vi "Make 2D Voltage Calibration Plots.vi"() -> ()   [LabVIEW 2019]
uses:
  <vilib>/Utility/file.llb/Read Delimited Spreadsheet (I64).vi
  <vilib>/Utility/file.llb/Write Delimited Spreadsheet (I64).vi
panel:
  out "Mask B Voltage vs. Mask A Voltage":i64[][](graph)
  in  "Pixel to Plot":i32
  in  "Pixel Data":path
  in  "Folder to save Pixel data":path
  in  "Starting Pixel":dbl
  in  "Starting Mask B Voltage":dbl
  in  "Ending Mask B Voltage":dbl
  in  "Current Mask B Voltage":dbl
  in  "Step Mask B Voltage":dbl
  in  "Generate Files (Px vs. Voltage)":bool
  in  "Ending Pixel":dbl
  in  "Current Pixel":dbl
  in  "Step":dbl
  in  "Folder of .txt 1D Calibration Files":path
  in  "Plot":bool
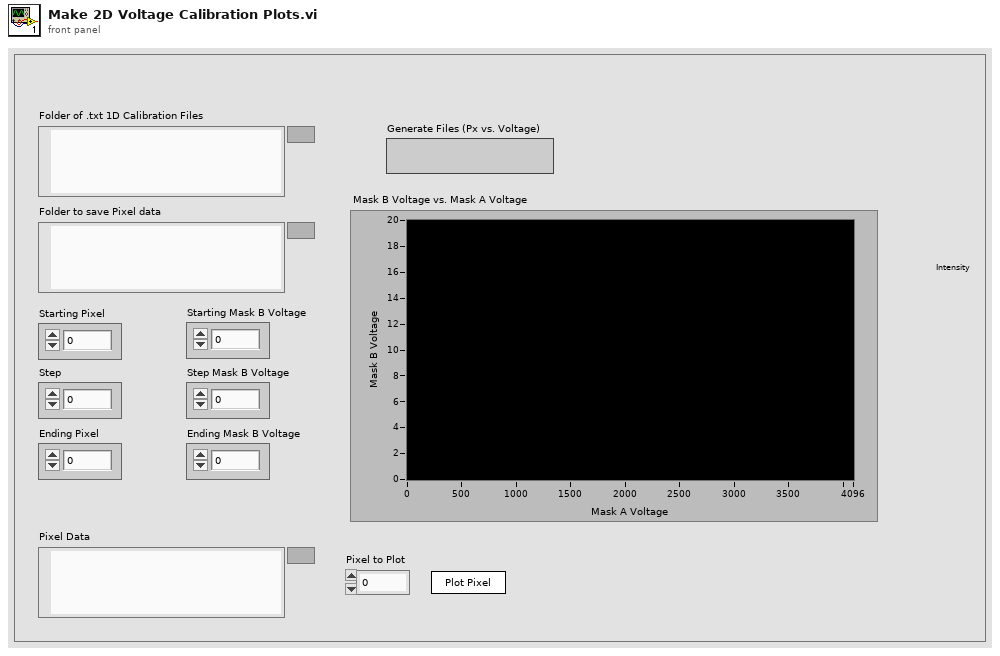
[diagram p1: front panel]
types:
  T1 = enum32{"Invalid", "Standard", "Closed", "Hidden", "Minimized", "Maximized"}
  T2 = enum32{"invalid app kind", "Development System", "Run Time System", "Student Edition", "Embedded LabVIEW", "Evaluation", "Custom"}
  T3 = enum16{"open", "replace", "create", "open or create", "replace or create", "replace or create with confirmation"}
  T4 = cluster{"Core":cluster{"Current VI Reference":refnum<vi>, "Close Panel on Exit?":bool}, "Starting Pixel":dbl, "Step":dbl, "Ending Pixel":dbl, "Current Pixel":dbl, "Starting Mask B Voltage":dbl, "Step Mask B Voltage":dbl, "Ending Mask B Voltage":dbl, "Current Mask B Voltage":dbl}
  T5 = cluster{"Current VI Reference":refnum<vi>, "Close Panel on Exit?":bool}
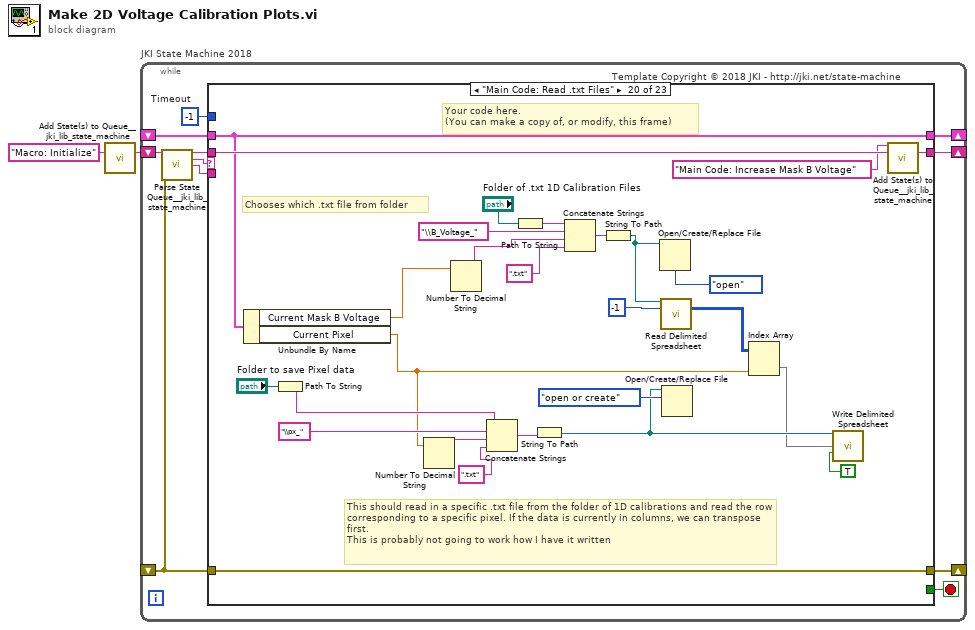
[diagram p0: block diagram]
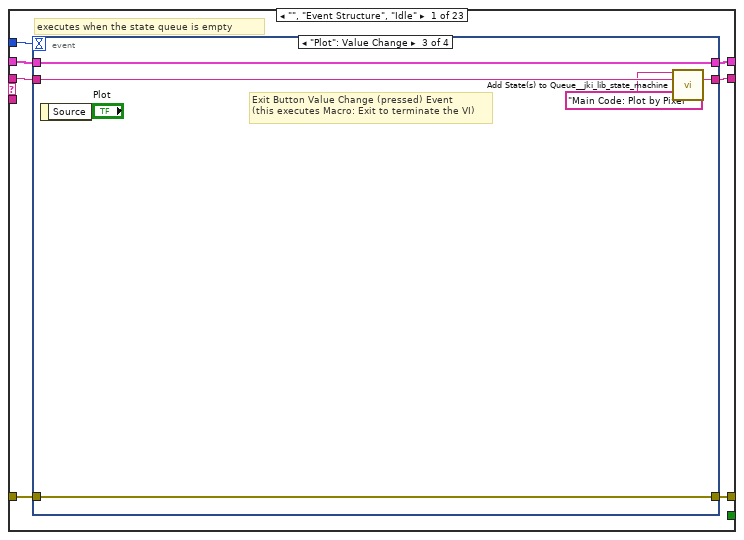
[diagram p2: hidden frame]
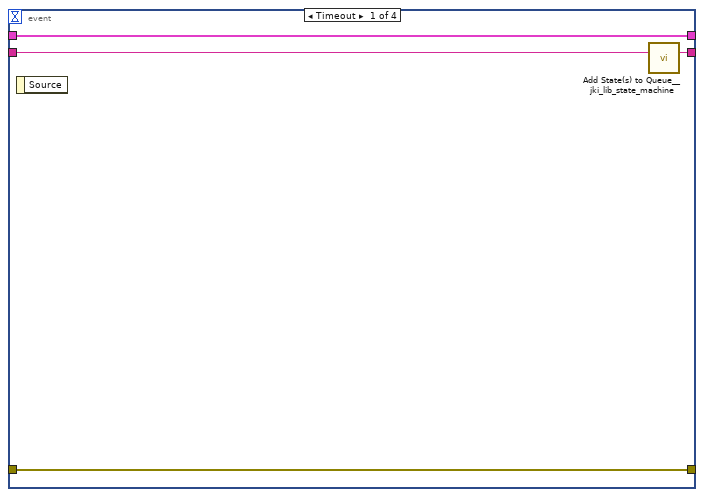
[diagram p3: hidden frame]
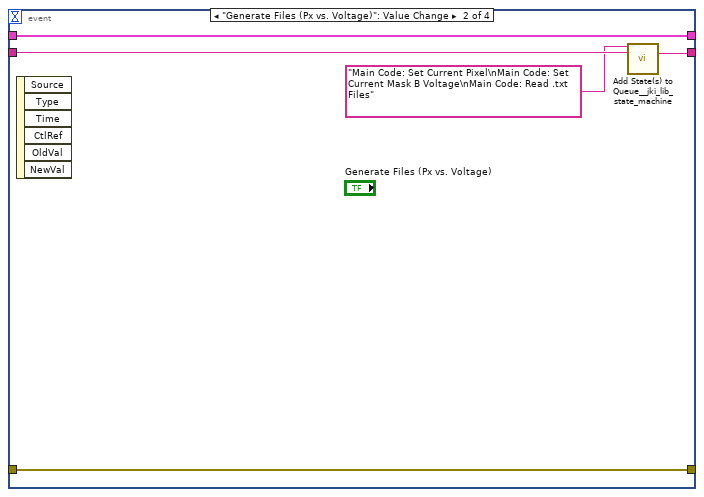
[diagram p4: hidden frame]
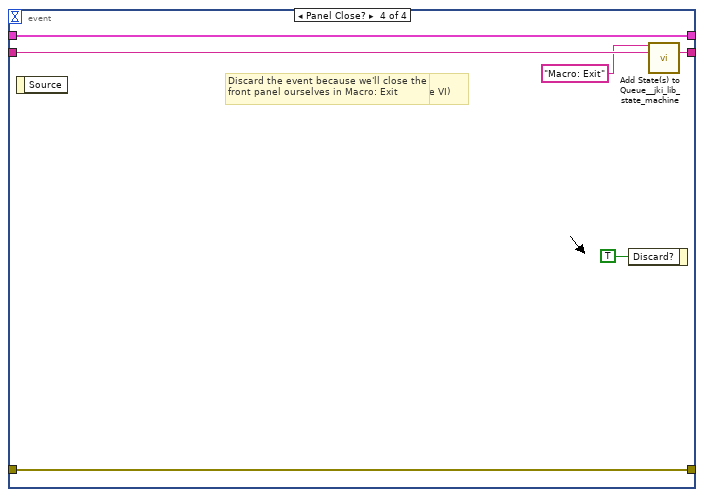
[diagram p5: hidden frame]
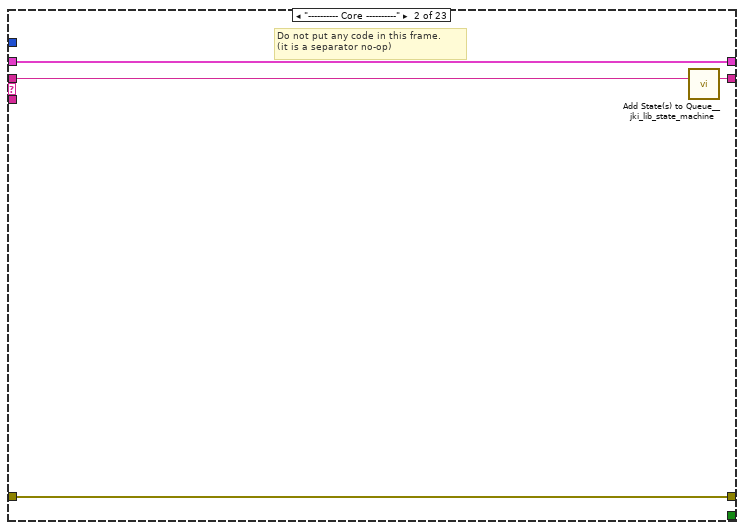
[diagram p6: hidden frame]
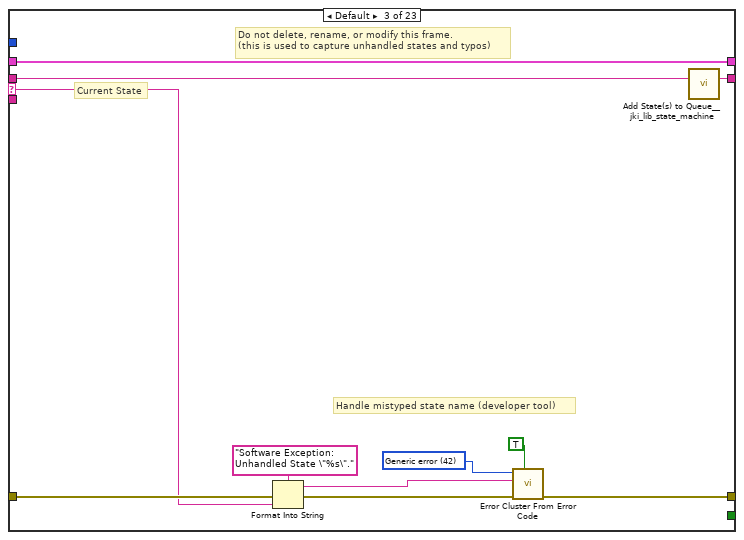
[diagram p7: hidden frame]
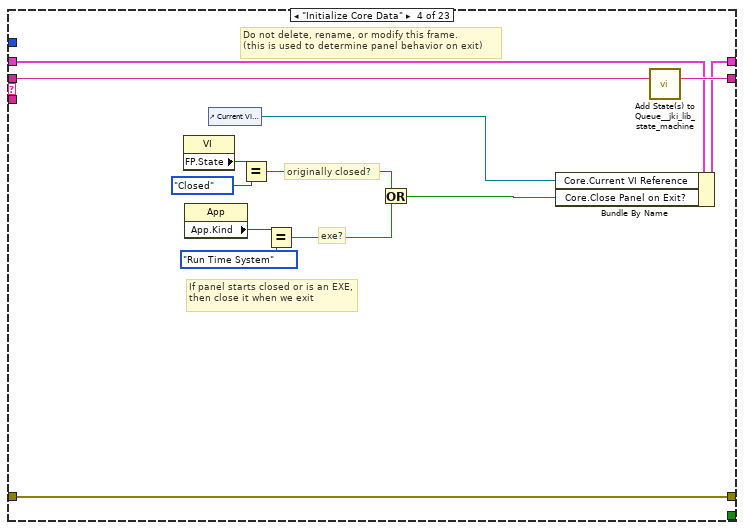
[diagram p8: hidden frame]
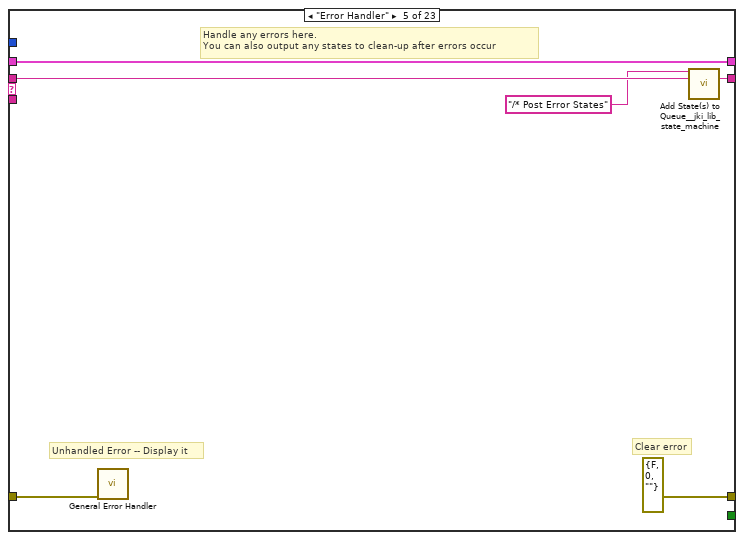
[diagram p9: hidden frame]
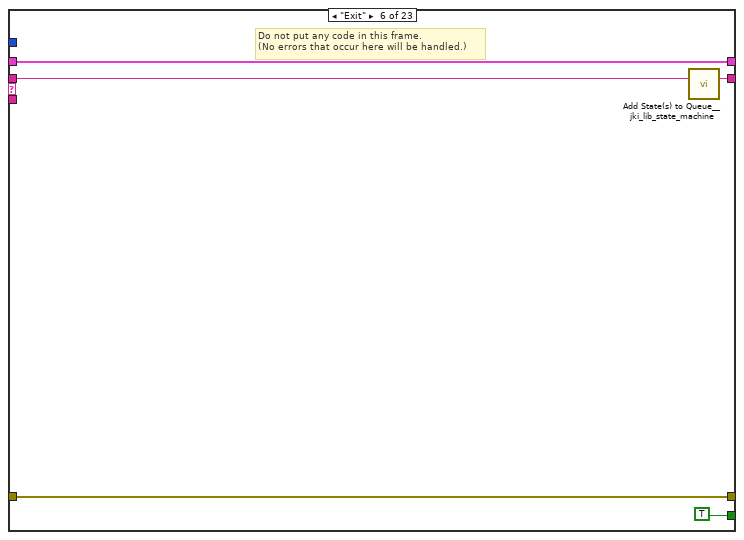
[diagram p10: hidden frame]
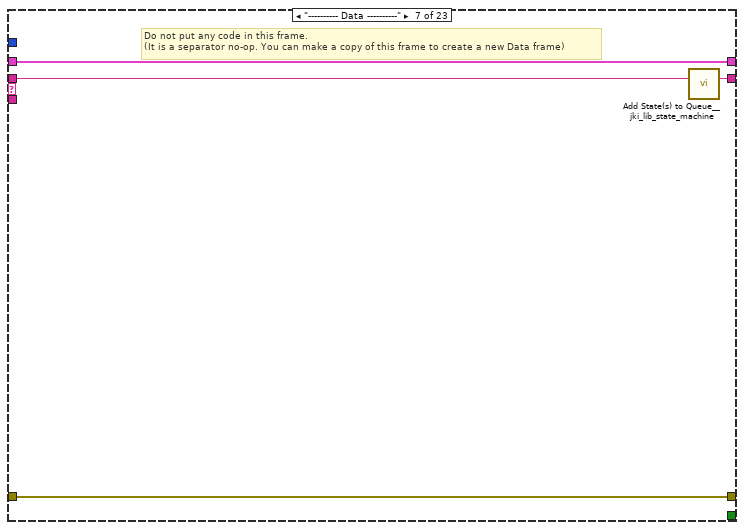
[diagram p11: hidden frame]
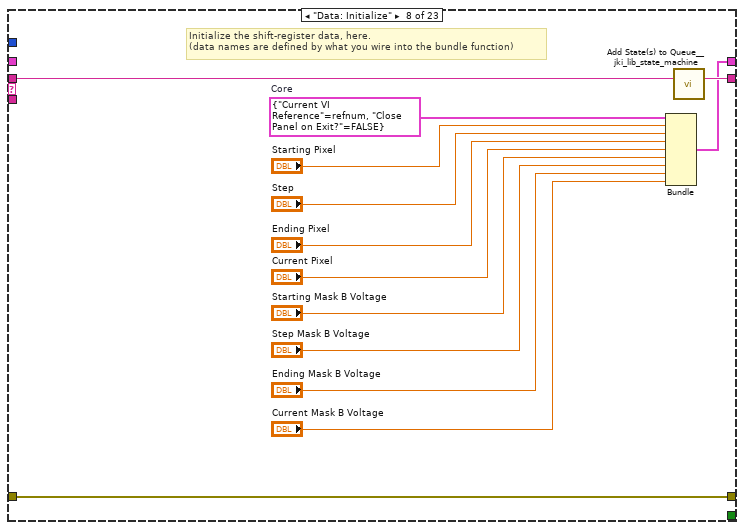
[diagram p12: hidden frame]
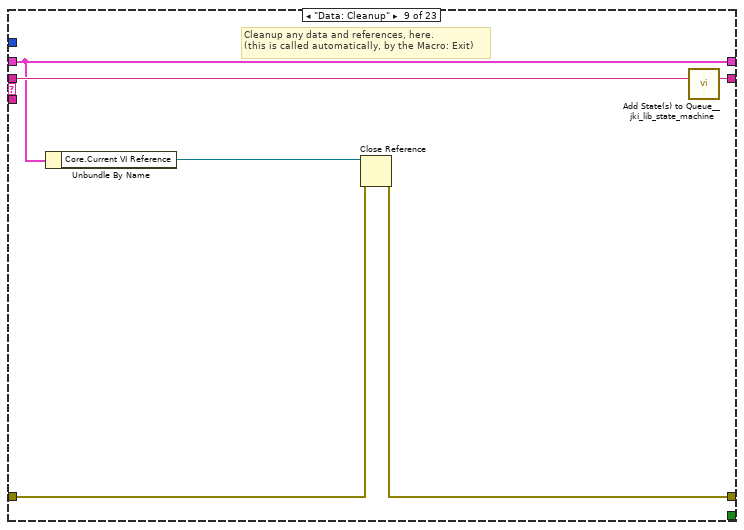
[diagram p13: hidden frame]
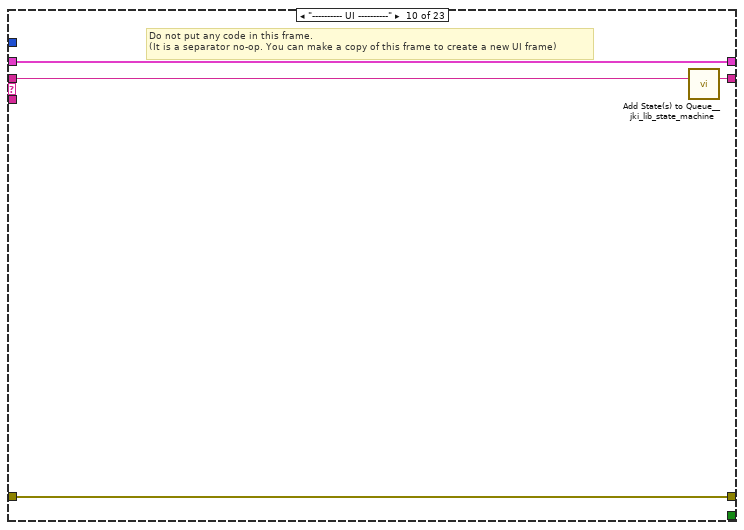
[diagram p14: hidden frame]
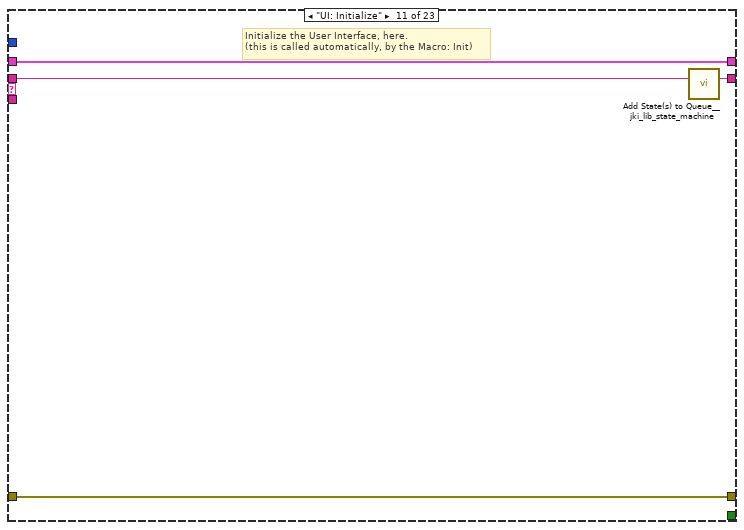
[diagram p15: hidden frame]
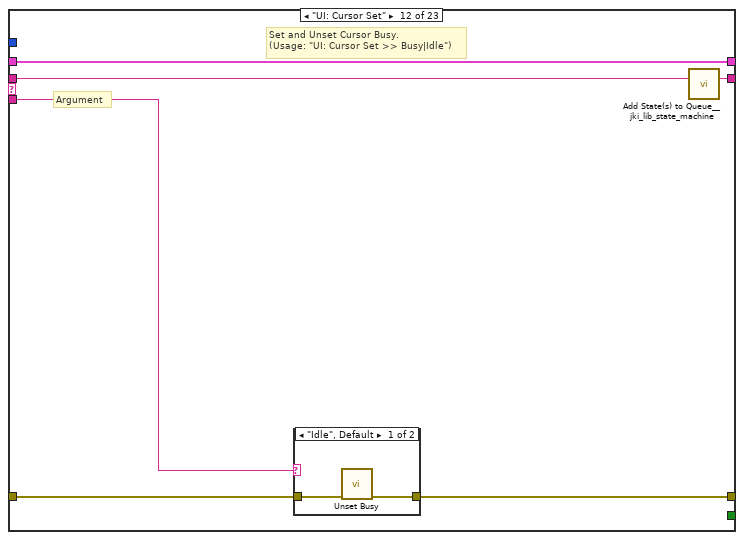
[diagram p16: hidden frame]
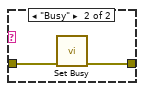
[diagram p17: hidden frame]
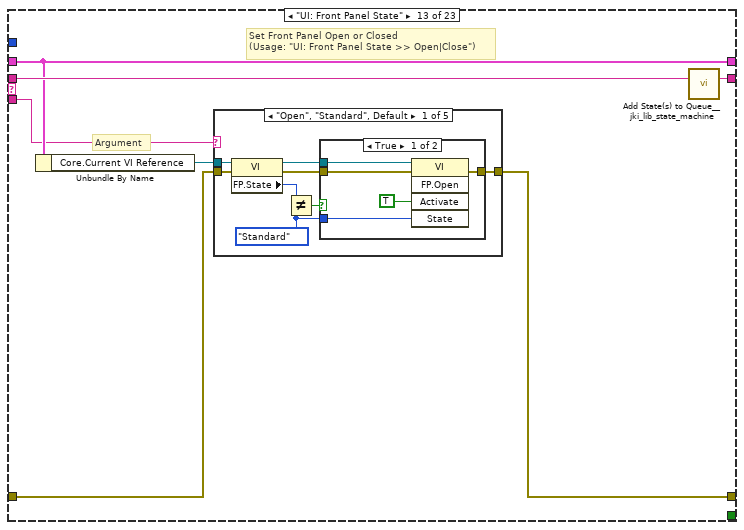
[diagram p18: hidden frame]
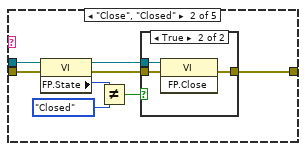
[diagram p20: hidden frame]
diagram:
  n1 = call <vilib>:"Add State(s) to Queue__jki_lib_state_machine.vi"("State(s) in (\"\")"="Macro: Initialize") -> ("States Out"=w2:string)  [unwired: 14 in]
  n2 = while "JKI State Machine 2018" {
    shift-right: [w6] -> _
    shift-left: _ -> [w5]
    shift-right: [w9] -> _
    shift-left: _ -> [w3]
    shift-right: [w8] -> _
    shift-left: w2 -> [w10]
    stop <- w7 stop-if-true
    w4 = -1  # Timeout
    # "Template Copyright © 2018 JKI - http://jki.net/state-machine"
    n3 = call <vilib>:"Parse State Queue__jki_lib_state_machine.vi"("State Queue"=w10, "Error In (no error)"=w3) -> ("Remaining States"=w12:string, "Current State"=w13:string, "Arguments"=w11:string)  [unwired: 11 in]
    n4 = case shown="\"Main Code: Read .txt Files\"" w13 {
      selector: w13 -> [_ _ w45 _ _ _ _ _ _ _ _ _ _ _ _ _ _ _ _ _ _ _ _]
      tunnel: w12 -> [w20 w44 w49 w68 w74 w79 w83 w96 w102 w106 w110 w116 w127 w196 w201 w211 w215 w221 w227 w254 w265 w285 w310]
      tunnel: w11 -> [_ _ _ _ _ _ _ _ _ _ _ w111 w121 _ _ _ _ _ _ _ _ _ _]
      tunnel: w5 -> [w18 w41 w47 w61 w71 w77 w80 _ w97 w103 w108 w114 w123 w193 w198 w208 w212 w218 w224 w243 w257 w278 w307]
      tunnel: [w17 w42 w51 w65 errorcluster {"status"=FALSE, "code"=0, "source"=""} ("error out") w76 w81 w93 w98 w104 w107 w112 w124 w194 w199 w209 w213 w219 w225 w252 w263 w283 w308] -> w9
      tunnel: w3 -> [w16 w42 w50 w65 w70 w76 w81 w93 w99 w104 w107 w113 w125 w194 w199 w209 w213 w219 w225 w252 w263 w283 w308]
      tunnel: [w19 w43 w48 w67 w73 w78 w82 w95 w101 w105 w109 w115 w126 w195 w200 w210 w214 w220 w226 w253 w264 w284 w309] -> w8
      tunnel: [_ _ _ _ _ TRUE _ _ _ _ _ _ _ _ _ _ _ _ _ _ _ _ _] -> w7
      tunnel: [w15 w41 w47 w66 w71 w77 w80 w94 w97 w103 w108 w114 w123 w193 w198 w208 w212 w217 w223 w243 w256 w277 w307] -> w6
      tunnel: w4 -> [w14 _ _ _ _ _ _ _ _ _ _ _ _ _ _ _ _ _ _ _ _ _ _]
      frame "", "Event Structure", "Idle" {
        # "executes when the state queue is empty"
        n5 = event shown="[2] \"Plot\": Value Change" {
          selector: _ -> [_ _ _ _]
          dyn-events: _ -> [_ _ _ _]
          timeout: w14 -> [_ _ _ _]
          tunnel: w20 -> [w24 w27 w34 w40]
          tunnel: [w23 w26 w33 w39] -> w19
          tunnel: w18 -> [w21 w28 w31 w37]
          tunnel: [w22 w29 w32 w38] -> w17
          tunnel: w16 -> [w22 w29 w32 w38]
          tunnel: [w21 w28 w31 w37] -> w15
          event Timeout {
            n6 = event-data() -> ()  [unwired: 1 in, 1 out]
            n7 = call <vilib>:"Add State(s) to Queue__jki_lib_state_machine.vi"("State(s) in (\"\")"=w24) -> ("States Out"=w23:string)  [unwired: 14 in]
          }
          event "Generate Files (Px vs. Voltage)": Value Change {
            n8 = event-data() -> ()  [unwired: 1 in, 6 out]
            n9 = call <vilib>:"Add State(s) to Queue__jki_lib_state_machine.vi"("State(s) in Front (\"\")"="Main Code: Set Current Pixel\nMain Code: Set Current Mask B Voltage\nMain Code: Read .txt Files" ("State(s) in Front (\"\")"), "State(s) in (\"\")"=w27) -> ("States Out"=w26:string)  [unwired: 13 in]
          }
          event "Plot": Value Change {
            # "Exit Button Value Change (pressed) Event\n(this executes Macro: Exit to terminate the VI)"
            n10 = event-data() -> ()  [unwired: 1 in, 1 out]
            n11 = call <vilib>:"Add State(s) to Queue__jki_lib_state_machine.vi"("State(s) in Front (\"\")"="Main Code: Plot by Pixel", "State(s) in (\"\")"=w34) -> ("States Out"=w33:string)  [unwired: 13 in]
          }
          event Panel Close? {
            # "Discard the event because we'll close the front panel ourselves in Macro: Exit"
            # "Close Panel button (pressed) Event\n(this executes Macro: Exit to terminate the VI)"
            n12 = event-data() -> ()  [unwired: 1 in, 1 out]
            n13 = event-data("Discard?"=TRUE) -> ()  [unwired: 1 in, 1 out]
            n14 = call <vilib>:"Add State(s) to Queue__jki_lib_state_machine.vi"("State(s) in Front (\"\")"="Macro: Exit", "State(s) in (\"\")"=w40) -> ("States Out"=w39:string)  [unwired: 13 in]
          }
        }
      }
      frame "---------- Core ----------" {
        # "Do not put any code in this frame.\n(it is a separator no-op)"
        n15 = call <vilib>:"Add State(s) to Queue__jki_lib_state_machine.vi"("State(s) in (\"\")"=w44) -> ("States Out"=w43:string)  [unwired: 14 in]
      }
      frame Default {
        w54 = 42 items=["No error", "Argument error", "Memory is full", "Out of zone", "End of file", "File already open", "Generic file I/O error", "File not found", "File permission error", "Disk is full", "Duplicate path", "Too many files open", "System feature not enabled", "Resource file not found", "Cannot add resource", "Resource not found", "Image not found", "Image memory error", "Pen does not exist", "Config type invalid", "Config token not found", "Config parse error", "Config memory error", "Bad external code format", "Bad external code offset", "External code not present", "Null window", "Destroy window error", "Null menu", "Print aborted", "Bad print record", "Print driver error", "Windows error during printing", "Memory error during printing", "Print dialog error", "Generic print error", "Invalid device refnum", "Device not found", "Device parameter error", "Device unit error", "Cannot open device", "Device call aborted", "Generic error", "Cancelled by user", "Object ID too low", "Object ID too high", "Object not in heap", "Unknown heap", "Unknown object (invalid DefProc)", "Unknown object (DefProc not in table)", "Message out of range", "Invalid (null) method", "Unknown message", "Manager call not supported", "Bad address", "Network operation in progress", "Network operation timed out", "Connection is busy", "Network attribute not supported", "Network error", "Address in use", "System out of memory", "Connection aborted", "Connection refused", "Not connected", "Already connected", "Connection closed", "Initialization error (interapplication manager)", "Bad occurrence", "Wait on unbound occurrence handler", "Occurrence queue overflow", "Datalog type conflict", "Unused", "Unrecognized type (interapplication manager)", "Memory corrupt", "Failed to make temporary DLL", "Old CIN version", "Drag socket not found", "Failed to load drop-object", "Failed to register OLE object", "Failed to release OLE object", "Format specifier type mismatch", "Unknown format specifier", "Too few format specifiers", "Too many format specifiers", "Scan failed", "Newer CIN version", "Error converting to variant", "Runtime menu error", "Password tampered", "Variant attribute not found", "Incompatible variant data type", "Event data is not available", "Event Store is not present", "Occurrence is not found", "Event Queue is not created", "Event info is not available", "Refnum passed is NULL", "Error retrieving Class GUID", "Error retrieving CoClass GUID", "Error retrieving TypeLib GUID.", "Bad built application magic bytes.", "Specific driver is different from the specific driver associated with the Logical Name.", "There is no session opened to the class driver.", "Max Error", "MAX - Error with config objects", "MAX - Error loading configuration", "MAX - Group not supported"]
        # "Current State"
        # "Do not delete, rename, or modify this frame.\n(this is used to capture unhandled states and typos)"
        # "Handle mistyped state name (developer tool)"
        n16 = Format Into String(format string="Software Exception: Unhandled State \"%s\"." ("message"), error in=w50, w45) -> (resulting string=w53:string, error out=w52:errorcluster)  [unwired: 1 in]
        n17 = call <vilib>:"Error Cluster From Error Code.vi"("show call chain? (False)"=TRUE, "error in (no error)"=w52, "error message (\"\")"=w53, "error code (0)"=w54) -> ("error out"=w51:errorcluster)  [unwired: 5 in]
        n18 = call <vilib>:"Add State(s) to Queue__jki_lib_state_machine.vi"("State(s) in (\"\")"=w49) -> ("States Out"=w48:string)  [unwired: 14 in]
      }
      frame "Initialize Core Data" {
        # "Do not delete, rename, or modify this frame.\n(this is used to determine panel behavior on exit)"
        # "originally closed?"
        # "exe?"
        # "If panel starts closed or is an EXE, then close it when we exit"
        n19 = property class="VI"() -> ("FP.State"=w58:T1)  [unwired: 2 in, 2 out]
        n20 = property class="App"() -> ("App.Kind"=w64:T2)  [unwired: 2 in, 2 out]
        n21 = control-ref of="Current VI Reference"() -> (w59:refnum<vi>)
        n22 = Equal?(x=w58, y=T1."Closed" ("Front Panel Window:State")) -> (x = y?=w56:bool)
        n23 = Equal?(x=w64, y=T2."Run Time System" ("Application:Kind")) -> (x = y?=w62:bool)
        n24 = Or(x=w56, y=w62) -> (x .or. y?=w60:bool)
        n25 = Bundle By Name(cluster=w61, "Core.Current VI Reference"=w59, "Core.Close Panel on Exit?"=w60) -> (w66:T4)
        n26 = call <vilib>:"Add State(s) to Queue__jki_lib_state_machine.vi"("State(s) in (\"\")"=w68) -> ("States Out"=w67:string)  [unwired: 14 in]
      }
      frame "Error Handler" {
        # "Unhandled Error -- Display it"
        # "Handle any errors here.\nYou can also output any states to clean-up after errors occur"
        # "Clear error"
        n27 = call <vilib>:"General Error Handler.vi"("error in (no error)"=w70) -> ()  [unwired: 10 in, 5 out]
        n28 = call <vilib>:"Add State(s) to Queue__jki_lib_state_machine.vi"("State(s) in Front (\"\")"="/* Post Error States", "State(s) in (\"\")"=w74) -> ("States Out"=w73:string)  [unwired: 13 in]
      }
      frame "Exit" {
        # "Do not put any code in this frame.\n(No errors that occur here will be handled.)"
        n29 = call <vilib>:"Add State(s) to Queue__jki_lib_state_machine.vi"("State(s) in (\"\")"=w79) -> ("States Out"=w78:string)  [unwired: 14 in]
      }
      frame "---------- Data ----------" {
        # "Do not put any code in this frame.\n(It is a separator no-op. You can make a copy of this frame to create a new Data frame)"
        n30 = call <vilib>:"Add State(s) to Queue__jki_lib_state_machine.vi"("State(s) in (\"\")"=w83) -> ("States Out"=w82:string)  [unwired: 14 in]
      }
      frame "Data: Initialize" {
        w92 = T5 {"Current VI Reference"=refnum, "Close Panel on Exit?"=FALSE}  # Core
        # "Initialize the shift-register data, here.\n(data names are defined by what you wire into the bundle function)"
        n31 = Bundle("Core"=w92, "Starting Pixel"="Starting Pixel", "Step"="Step", "Ending Pixel"="Ending Pixel", "Current Pixel"="Current Pixel", "Starting Mask B Voltage"="Starting Mask B Voltage", "Step Mask B Voltage"="Step Mask B Voltage", "Ending Mask B Voltage"="Ending Mask B Voltage", "Current Mask B Voltage"="Current Mask B Voltage") -> (w94:T4)  [unwired: 1 in]
        n32 = call <vilib>:"Add State(s) to Queue__jki_lib_state_machine.vi"("State(s) in (\"\")"=w96) -> ("States Out"=w95:string)  [unwired: 14 in]
      }
      frame "Data: Cleanup" {
        # "Cleanup any data and references, here.\n(this is called automatically, by the Macro: Exit)"
        n33 = Unbundle By Name(w97) -> ("Core.Current VI Reference"=w100:refnum<vi>)
        n34 = Close Reference(reference=w100, error in (no error)=w99) -> (error out=w98:errorcluster)
        n35 = call <vilib>:"Add State(s) to Queue__jki_lib_state_machine.vi"("State(s) in (\"\")"=w102) -> ("States Out"=w101:string)  [unwired: 14 in]
      }
      frame "---------- UI ----------" {
        # "Do not put any code in this frame.\n(It is a separator no-op. You can make a copy of this frame to create a new UI frame)"
        n36 = call <vilib>:"Add State(s) to Queue__jki_lib_state_machine.vi"("State(s) in (\"\")"=w106) -> ("States Out"=w105:string)  [unwired: 14 in]
      }
      frame "UI: Initialize" {
        # "Initialize the User Interface, here.\n(this is called automatically, by the Macro: Init)"
        n37 = call <vilib>:"Add State(s) to Queue__jki_lib_state_machine.vi"("State(s) in (\"\")"=w110) -> ("States Out"=w109:string)  [unwired: 14 in]
      }
      frame "UI: Cursor Set" {
        # "Argument"
        # "Set and Unset Cursor Busy.\n(Usage: \"UI: Cursor Set >> Busy|Idle\")"
        n38 = case shown="\"Idle\", Default" w111 {
          tunnel: w113 -> [w118 w120]
          tunnel: [w117 w119] -> w112
          frame "Idle", Default {
            n39 = call <vilib>:"Unset Busy.vi"("error in (no error)"=w118) -> ("error out"=w117:errorcluster)  [unwired: 10 in]
          }
          frame "Busy" {
            n40 = call <vilib>:"Set Busy.vi"("error in (no error)"=w120) -> ("error out"=w119:errorcluster)  [unwired: 9 in, 1 out]
          }
        }
        n41 = call <vilib>:"Add State(s) to Queue__jki_lib_state_machine.vi"("State(s) in (\"\")"=w116) -> ("States Out"=w115:string)  [unwired: 14 in]
      }
      frame "UI: Front Panel State" {
        # "Argument"
        # "Set Front Panel Open or Closed\n(Usage: \"UI: Front Panel State >> Open|Close\")"
        n42 = Unbundle By Name(w123) -> ("Core.Current VI Reference"=w122:refnum<vi>)
        n43 = case shown="\"Open\", \"Standard\", Default" w121 {
          tunnel: w125 -> [w133 w148 w159 w172 w185]
          tunnel: [w135 w149 w161 w174 w187] -> w124
          tunnel: w122 -> [w134 w146 w160 w173 w186]
          frame "Open", "Standard", Default {
            w128 = T1."Standard" ("State")
            n44 = property class="VI"(reference=w134, error in=w133) -> (reference out=w131:refnum<vi>, error out=w132:errorcluster, "FP.State"=w130:T1)
            n45 = Not Equal?(x=w130, y=w128) -> (x != y?=w129:bool)
            n46 = case shown="True" w129 {
              tunnel: [w139 w141] -> w135
              tunnel: w132 -> [w138 w141]
              tunnel: w131 -> [w137 _]
              tunnel: w128 -> [w136 _]
              frame True {
                n47 = invoke class="VI" method="FP.Open"(reference=w137, error in=w138, "Activate"=TRUE, "State"=w136) -> (error out=w139:errorcluster)  [unwired: 1 in, 4 out]
              }
              frame False {
              }
            }
          }
          frame "Close", "Closed" {
            n48 = property class="VI"(reference=w146, error in=w148) -> (reference out=w145:refnum<vi>, error out=w147:errorcluster, "FP.State"=w143:T1)
            n49 = Not Equal?(x=w143, y=T1."Closed" ("Front Panel Window:State")) -> (x != y?=w142:bool)
            n50 = case shown="True" w142 {
              tunnel: [w150 w153] -> w149
              tunnel: w147 -> [w150 w152]
              tunnel: w145 -> [_ w151]
              frame False {
              }
              frame True {
                n51 = invoke class="VI" method="FP.Close"(reference=w151, error in=w152) -> (error out=w153:errorcluster)  [unwired: 1 in, 2 out]
              }
            }
          }
          frame "Hidden", "Hide" {
            w154 = T1."Hidden" ("State")
            n52 = property class="VI"(reference=w160, error in=w159) -> (reference out=w157:refnum<vi>, error out=w158:errorcluster, "FP.State"=w156:T1)
            n53 = Not Equal?(x=w156, y=w154) -> (x != y?=w155:bool)
            n54 = case shown="True" w155 {
              tunnel: [w165 w166] -> w161
              tunnel: w158 -> [w164 w166]
              tunnel: w157 -> [w163 _]
              tunnel: w154 -> [w162 _]
              frame True {
                n55 = invoke class="VI" method="FP.Open"(reference=w163, error in=w164, "State"=w162) -> (error out=w165:errorcluster)  [unwired: 2 in, 4 out]
              }
              frame False {
              }
            }
          }
          frame "Minimize", "Minimized" {
            w167 = T1."Minimized" ("State")
            n56 = property class="VI"(reference=w173, error in=w172) -> (reference out=w170:refnum<vi>, error out=w171:errorcluster, "FP.State"=w169:T1)
            n57 = Not Equal?(x=w169, y=w167) -> (x != y?=w168:bool)
            n58 = case shown="True" w168 {
              tunnel: [w178 w179] -> w174
              tunnel: w171 -> [w177 w179]
              tunnel: w170 -> [w176 _]
              tunnel: w167 -> [w175 _]
              frame True {
                n59 = invoke class="VI" method="FP.Open"(reference=w176, error in=w177, "State"=w175) -> (error out=w178:errorcluster)  [unwired: 2 in, 4 out]
              }
              frame False {
              }
            }
          }
          frame "Maximize", "Maximized" {
            w180 = T1."Maximized" ("State")
            n60 = property class="VI"(reference=w186, error in=w185) -> (reference out=w183:refnum<vi>, error out=w184:errorcluster, "FP.State"=w182:T1)
            n61 = Not Equal?(x=w182, y=w180) -> (x != y?=w181:bool)
            n62 = case shown="True" w181 {
              tunnel: [w191 w192] -> w187
              tunnel: w184 -> [w190 w192]
              tunnel: w183 -> [w189 _]
              tunnel: w180 -> [w188 _]
              frame True {
                n63 = invoke class="VI" method="FP.Open"(reference=w189, error in=w190, "State"=w188) -> (error out=w191:errorcluster)  [unwired: 2 in, 4 out]
              }
              frame False {
              }
            }
          }
        }
        n64 = call <vilib>:"Add State(s) to Queue__jki_lib_state_machine.vi"("State(s) in (\"\")"=w127) -> ("States Out"=w126:string)  [unwired: 14 in]
      }
      frame "---------- Macro ----------" {
        # "Do not put any code in this frame.\n(It is a separator no-op. You can make a copy of this frame to create a new Macro frame)"
        n65 = call <vilib>:"Add State(s) to Queue__jki_lib_state_machine.vi"("State(s) in (\"\")"=w196) -> ("States Out"=w195:string)  [unwired: 14 in]
      }
      frame "Macro: Initialize" {
        w197 = "Data: Initialize\nInitialize Core Data\nUI: Initialize\nUI: Front Panel State >> Open"  # Data: Initialize Initialize Core Data UI: Initialize UI: Front Panel State >> Open
        # "Initialization Macro\n(This is called once, when the VI starts)"
        n66 = call <vilib>:"Add State(s) to Queue__jki_lib_state_machine.vi"("State(s) in Front (\"\")"=w197, "State(s) in (\"\")"=w201) -> ("States Out"=w200:string)  [unwired: 13 in]
      }
      frame "Macro: Exit" {
        # "Exit Macro\n(This is called once, when the VI exits)"
        n67 = Unbundle By Name(w208) -> ("Core.Close Panel on Exit?"=w207:bool)
        n68 = Select(t="UI: Front Panel State >> Close", s=w207, f="") -> (s? t:f=w204:string)
        n69 = call <vilib>:"Add State(s) to Queue__jki_lib_state_machine.vi"("State(s) in (\"\")"=w204, "State(s) at Back (\"\")"="Data: Cleanup\nExit") -> ("States Out"=w202:string)  [unwired: 13 in]
        n70 = call <vilib>:"Add State(s) to Queue__jki_lib_state_machine.vi"("State(s) in Front (\"\")"=w202, "State(s) in (\"\")"=w211) -> ("States Out"=w210:string)  [unwired: 13 in]
      }
      frame "---------- Main Code ----------" {
        # "Template Separator\n(You can make a copy of, or modify, this frame)"
        n71 = call <vilib>:"Add State(s) to Queue__jki_lib_state_machine.vi"("State(s) in (\"\")"=w215) -> ("States Out"=w214:string)  [unwired: 14 in]
      }
      frame "Main Code: Set Current Pixel" {
        # "This state is called once when the \"go\" button is hit so we use current pixel rather than changing starting pixel.\nCurrent pixel will not be seen or controlled by the user while starting pixel is. This removes some chance for error."
        # "Template Separator\n(You can make a copy of, or modify, this frame)"
        n72 = Unbundle By Name(w218) -> ("Starting Pixel"=w216:dbl)
        n73 = Bundle By Name(cluster=w218, "Current Pixel"=w216) -> (w217:T4)
        n74 = call <vilib>:"Add State(s) to Queue__jki_lib_state_machine.vi"("State(s) in (\"\")"=w221) -> ("States Out"=w220:string)  [unwired: 14 in]
      }
      frame "Main Code: Set Current Mask B Voltage" {
        # "This state is called once when the \"go\" button is hit so we use current pixel rather than changing starting pixel.\nCurrent pixel will not be seen or controlled by the user while starting pixel is. This removes some chance for error."
        # "Template Separator\n(You can make a copy of, or modify, this frame)"
        n75 = Unbundle By Name(w224) -> ("Starting Mask B Voltage"=w222:dbl)
        n76 = Bundle By Name(cluster=w224, "Current Mask B Voltage"=w222) -> (w223:T4)
        n77 = call <vilib>:"Add State(s) to Queue__jki_lib_state_machine.vi"("State(s) in (\"\")"=w227) -> ("States Out"=w226:string)  [unwired: 14 in]
      }
      frame "Main Code: Read .txt Files" {
        # "Chooses which .txt file from folder"
        # "This should read in a specific .txt file from the folder of 1D calibrations and read the row corresponding to a specific pixel. If the data is currently in columns, we can transpose first.\nThis is probably not going to work how I have it written"
        # "Your code here.\n(You can make a copy of, or modify, this frame)"
        n78 = Unbundle By Name(w243) -> ("Current Mask B Voltage"=w242:dbl, "Current Pixel"=w234:dbl)
        n79 = Path To String(path="Folder to save Pixel data") -> (string=w236:string)
        n80 = Number To Decimal String(number=w234) -> (decimal integer string=w233:string)  [unwired: 1 in]
        n81 = Number To Decimal String(number=w242) -> (decimal integer string=w247:string)  [unwired: 1 in]
        n82 = Concatenate Strings(w236, "\\px_", w233, ".txt") -> (w232:string)
        n83 = Path To String(path="Folder of .txt 1D Calibration Files") -> (string=w249:string)
        n84 = String To Path(string=w232) -> (path=w230:path)
        n85 = Concatenate Strings(w249, "\\B_Voltage_", w247, ".txt") -> (w248:string)
        n86 = String To Path(string=w248) -> (path=w245:path)
        n87 = Open/Create/Replace File(file path (use dialog)=w245, operation (0:open)=T3."open") -> ()  [unwired: 4 in, 3 out]
        n88 = call-poly <vilib>:"Read Delimited Spreadsheet.vi"("file path (dialog if empty)"=w245, "number of rows (all:-1)"=-1) -> ("all rows"=w238:i64[][])  [unwired: 8 in, 5 out]
        n89 = Open/Create/Replace File(file path (use dialog)=w230, operation (0:open)=T3."open or create") -> ()  [unwired: 4 in, 3 out]
        n90 = Index Array(array=w238, index (col)=w234) -> (element=w228:i64[])  [unwired: 1 in]
        n91 = call-poly <vilib>:"Write Delimited Spreadsheet.vi"("file path (dialog if empty)"=w230, "1D data"=w228, "append to file? (new file:F)"=TRUE ("transpose? (F)")) -> ()  [unwired: 11 in, 2 out]
        n92 = call <vilib>:"Add State(s) to Queue__jki_lib_state_machine.vi"("State(s) in Front (\"\")"="Main Code: Increase Mask B Voltage" ("State(s) in Front (\"\")"), "State(s) in (\"\")"=w254) -> ("States Out"=w253:string)  [unwired: 13 in]
      }
      frame "Main Code: Increase Mask B Voltage" {
        # "True: If not done with all mask B voltages, increase Mask B Voltage and call Read .txt Files to read same pixel from next .txt file.\nFalse: If done with all scanned mask B voltages, reset current mask B voltage to strarting mask B voltage and call Increase Pixel"
        # "Template Separator\n(You can make a copy of, or modify, this frame)"
        n93 = Unbundle By Name(w257) -> ("Starting Mask B Voltage"=w255:dbl, "Step Mask B Voltage"=w260:dbl, "Current Mask B Voltage"=w259:dbl, "Ending Mask B Voltage"=w262:dbl)
        n94 = Less?(x=w259, y=w262) -> (x < y?=w261:bool)
        n95 = case shown="True" w261 {
          tunnel: w260 -> [_ w275]
          tunnel: w259 -> [_ w274]
          tunnel: ["Main Code: Increase Pixel" ("State(s) in Front (\"\")") "Main Code: Read .txt Files" ("State(s) in Front (\"\")")] -> w258
          tunnel: w257 -> [w267 w272]
          tunnel: [w268 w270] -> w256
          tunnel: w255 -> [w266 _]
          frame False {
            n96 = Bundle By Name(cluster=w267, "Current Mask B Voltage"=w266) -> (w268:T4)
          }
          frame True {
            n97 = Add(x=w275, y=w274) -> (x+y=w271:dbl)
            n98 = Bundle By Name(cluster=w272, "Current Mask B Voltage"=w271) -> (w270:T4)
          }
        }
        n99 = call <vilib>:"Add State(s) to Queue__jki_lib_state_machine.vi"("State(s) in Front (\"\")"=w258, "State(s) in (\"\")"=w265) -> ("States Out"=w264:string)  [unwired: 13 in]
      }
      frame "Main Code: Increase Pixel" {
        # "True: If not done with user defined pixel range, increase pixel number and start reading files for all mask B voltages.\nFalse: If done with all pixels, finish reading files and go to idle. From here, the user can choose to plot any given pixel (I am not sure how to do this.)\nI want to automatically save the plot for each pixel as a .txt file. Once that is done, the user should be able to choose a pixel number and have the code read that file and plot the data. \nThe \"go\" button should transfer ALL data from pixel v mask A voltage for each mask B voltage to mask A voltage v mask B voltage for each pixel\nThe \"plot this pixel\" button should plot the pixel chosen by the user"
        # "Template Separator\n(You can make a copy of, or modify, this frame)"
        n100 = Unbundle By Name(w278) -> ("Step"=w280:dbl, "Current Pixel"=w279:dbl, "Ending Pixel"=w282:dbl)
        n101 = Less?(x=w279, y=w282) -> (x < y?=w281:bool)
        n102 = case shown="True" w281 {
          tunnel: w280 -> [_ w295]
          tunnel: w279 -> [w286 w294]
          tunnel: w278 -> [w288 w293]
          tunnel: [w289 w291] -> w277
          tunnel: ["Idle" ("State(s) in Front (\"\")") "Main Code: Read .txt Files" ("State(s) in Front (\"\")")] -> w276
          frame False {
            n103 = Bundle By Name(cluster=w288, "Current Pixel"=w286) -> (w289:T4)
          }
          frame True {
            n104 = Add(x=w295, y=w294) -> (x+y=w292:dbl)
            n105 = Bundle By Name(cluster=w293, "Current Pixel"=w292) -> (w291:T4)
          }
        }
        n106 = call <vilib>:"Add State(s) to Queue__jki_lib_state_machine.vi"("State(s) in Front (\"\")"=w276, "State(s) in (\"\")"=w285) -> ("States Out"=w284:string)  [unwired: 13 in]
      }
      frame "Main Code: Plot by Pixel" {
        # "Your code here.\n(You can make a copy of, or modify, this frame)"
        n107 = Path To String(path="Pixel Data") -> (string=w305:string)
        n108 = Number To Decimal String(number="Pixel to Plot") -> (decimal integer string=w303:string)  [unwired: 1 in]
        n109 = Concatenate Strings(w305, "\\px_", w303, ".txt") -> (w302:string)
        n110 = String To Path(string=w302) -> (path=w298:path)
        n111 = Open/Create/Replace File(file path (use dialog)=w298, operation (0:open)=T3."open") -> ()  [unwired: 4 in, 3 out]
        n112 = call-poly <vilib>:"Read Delimited Spreadsheet.vi"("file path (dialog if empty)"=w298, "transpose? (F)"=TRUE) -> ("all rows"=→"Mask B Voltage vs. Mask A Voltage":i64[][])  [unwired: 8 in, 5 out]
        n113 = call <vilib>:"Add State(s) to Queue__jki_lib_state_machine.vi"("State(s) in (\"\")"=w310) -> ("States Out"=w309:string)  [unwired: 14 in]
      }
    }
  }
